vi "Load.vi"   [LabVIEW 2021]
uses:
  Child.lvclass
  C:/PPLs/Decorating-Template-Method-with-Interfaces/Template Method with Interfaces/Interface/Interface.lvclass
  Interface/Interface.lvclass
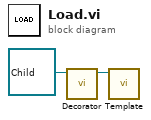
[diagram p0: block diagram]
diagram:
  n1 = call "Decorator.vi"("Child in"=refnum<class "Child.lvclass"> refnum ("Child.lvclass")) -> ("Child out"=w1:refnum<class "Child.lvclass">)  [unwired: 9 in, 1 out]
  n2 = call "Template.vi"("Interface in"=w1) -> ()  [unwired: 11 in]
